vi "Initialize Settings File.vi"() -> (0 "error out":errorcluster, 3 "named_positions":T1[](array[typedef]))   [LabVIEW 2020, in "Manipulator.lvlib"]
uses:
  Manipulator.lvlib
  Named Position.ctl
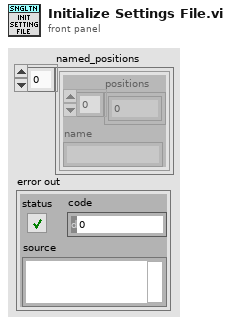
[diagram p1: front panel]
types:
  T1 = typedef "Manipulator.lvlib/Named Position.ctl" = cluster{"positions":dbl[], "name":string}
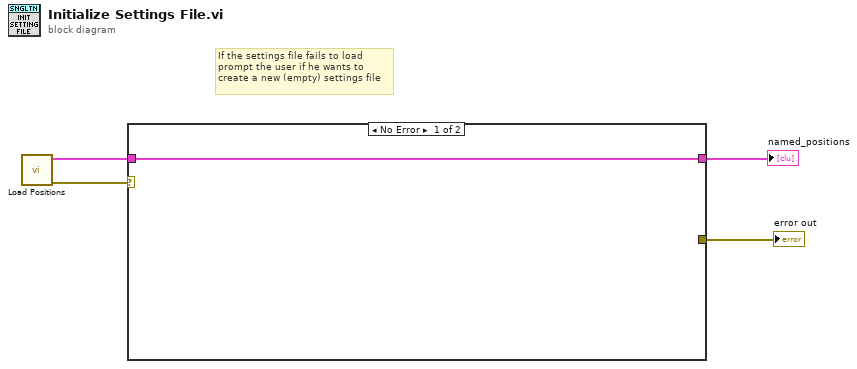
[diagram p0: block diagram]
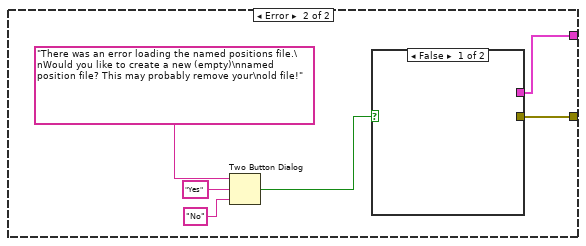
[diagram p2: hidden frame]
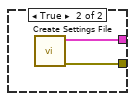
[diagram p3: hidden frame]
diagram:
  # "If the settings file fails to load\nprompt the user if he wants to\ncreate a new (empty) settings file"
  n1 = call "Load Positions.vi"() -> ("error out"=w3:errorcluster, "positions"=w4:T1[])  [unwired: 10 in]
  n2 = case shown="No Error" w3 {
    tunnel: w4 -> [w5 _]
    tunnel: [w5 w6] -> w1
    tunnel: [_ w7] -> w2
    frame No Error {
    }
    frame Error {
      n3 = Two Button Dialog(message="There was an error loading the named positions file.\nWould you like to create a new (empty)\nnamed position file? This may probably remove your\nold file!", 1:"No" ("F button name (\"Cancel\")"), 2:"Yes" ("T button name (\"OK\")")) -> (T button?=w8:bool)
      n4 = case shown="False" w8 {
        tunnel: [_ w13] -> w7
        tunnel: [_ w12] -> w6
        frame False {
        }
        frame True {
          n5 = call "Create Settings File.vi"() -> ("error out"=w13:errorcluster, "named_positions"=w12:T1[])  [unwired: 10 in]
        }
      }
    }
  }
  "named_positions" <- w1
  "error out" <- w2
